vi "DownSampleiRF (SubVI).vi"(11 "ArrayIn":dbl[](array[numeric])) -> (3 "ArrayOut":dbl[](array[numeric]))   [LabVIEW 2021]
uses:
  <vilib>/Analysis/baseanly.llb/Mean (DBL).vi
  <vilib>/Analysis/NI_AALBase.lvlib
panel:
  out "Waveform Graph":dbl[](graph)
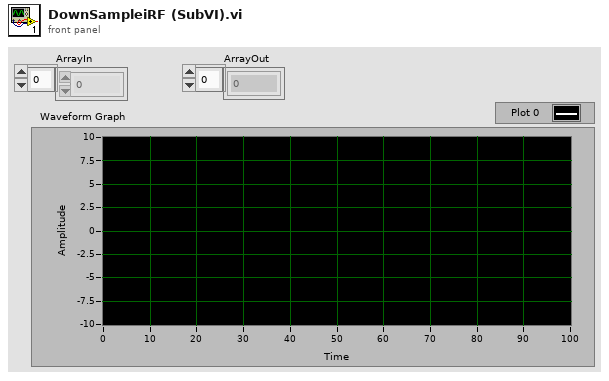
[diagram p1: front panel]
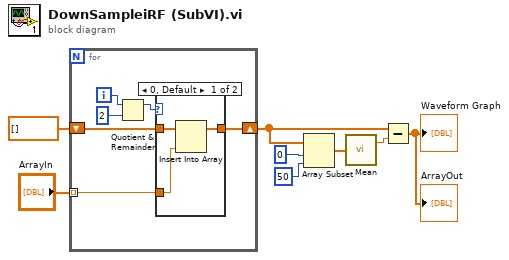
[diagram p0: block diagram]
diagram:
  n1 = for {
    tunnel: "ArrayIn" -> [w10] mode=indexing
    shift-right: [w9] -> w3
    shift-left: dbl[] [] -> [w11]
    i -> [w14]
    n2 = Quotient & Remainder(x=w14, y=2) -> (x-y*floor(x/y)=w12:i32)  [unwired: 1 out]
    n3 = case shown="0, Default" w12 {
      tunnel: w11 -> [w17 w18]
      tunnel: w10 -> [w16 _]
      tunnel: [w15 w18] -> w9
      frame 0, Default {
        n4 = Insert Into Array(array=w17, new element=w16) -> (w15:dbl[])  [unwired: 1 in]
      }
      frame 1 {
      }
    }
  }
  n5 = Array Subset(array=w3, index=0, length=50) -> (w4:dbl[])
  n6 = call-poly <vilib>:"Mean.vi"("X"=w4) -> ("mean"=w2:dbl)  [unwired: 1 out]
  n7 = Subtract(x=w3, y=w2) -> (x-y=→"ArrayOut" →"Waveform Graph":dbl[])
